vi "PH_PSDBWriter.write Dataset.vi"(1 "PSDB Credentials":T1={"PW"="N/A", "ID"="N/A", "DS"="N/A"}, 2 "Shot #":i32, 3 "Instance ID":i32, 4 "Data to write to PSDB":T2, 5 "error in (no error)":errorcluster) -> (19 "error out":errorcluster)   [LabVIEW 2014, in "PH_PSDBWriter.lvlib"]
uses:
  PH_PSDBWriter.lvlib
  PH_PSDBWriter.PSDB Dataset.ctl
  PH_PSDBWriter.2D dataset.ctl
  CSlibraries-extern/psdb_lv/PSDB_AxisDescription.ctl
  PH_PSDBWriter.Boolean dataset.ctl
  PH_PSDBWriter.Image dataset.ctl
  <vilib>/vision/Image Controls.llb/IMAQ Image.ctl
  PH_PSDBWriter.Numeric dataset.ctl
  PH_PSDBWriter.String dataset.ctl
  PH_Common/Connection/PH_Connection.PSDB Credentials.ctl
  CSlibraries-extern/psdb_lv/PSDB_SetInstanceValue(2dData).vi
  CSlibraries-extern/psdb_lv/PSDB_SetInstanceValue(Boolean).vi
  CSlibraries-extern/psdb_lv/PSDB_SetInstanceValue(Image).vi
  CSlibraries-extern/psdb_lv/PSDB_SetInstanceValue(Numeric).vi
  CSlibraries-extern/psdb_lv/PSDB_SetInstanceValue(String).vi
  CSlibraries-extern/psdb_lv/PSDB.lvlib
  PH_Common/PH_Common.lvlib
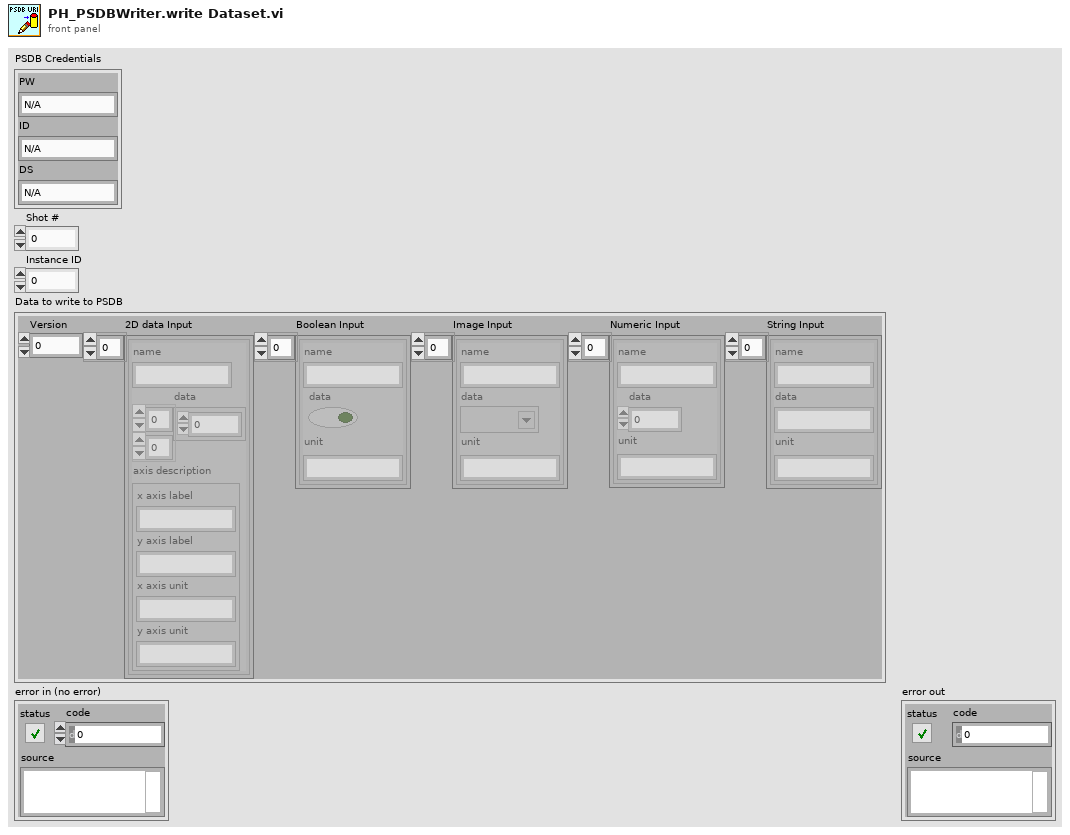
[diagram p1: front panel]
types:
  T1 = typedef "PH_Common.lvlib/PH_Connection.PSDB Credentials.ctl" = cluster{"PW":string, "ID":string, "DS":string}
  T2 = typedef "PH_PSDBWriter.lvlib/PH_PSDBWriter.PSDB Dataset.ctl" = cluster{"Version":i32, "2D data Input":T3[], "Boolean Input":T5[], "Image Input":T6[], "Numeric Input":T8[], "String Input":T9[]}
  T3 = typedef "PH_PSDBWriter.lvlib/PH_PSDBWriter.2D dataset.ctl" = cluster{"name":string, "data":dbl[][], "axis description":T4}
  T4 = typedef "PSDB.lvlib/PSDB_AxisDescription.ctl" = cluster{"x axis label":string, "y axis label":string, "x axis unit":string, "y axis unit":string}
  T5 = typedef "PH_PSDBWriter.lvlib/PH_PSDBWriter.Boolean dataset.ctl" = cluster{"name":string, "data":bool, "unit":string}
  T6 = typedef "PH_PSDBWriter.lvlib/PH_PSDBWriter.Image dataset.ctl" = cluster{"name":string, "data":T7, "unit":string}
  T7 = typedef "IMAQ Image.ctl" = refnum<image>
  T8 = typedef "PH_PSDBWriter.lvlib/PH_PSDBWriter.Numeric dataset.ctl" = cluster{"name":string, "data":dbl, "unit":string}
  T9 = typedef "PH_PSDBWriter.lvlib/PH_PSDBWriter.String dataset.ctl" = cluster{"name":string, "data":string, "unit":string}
  T10 = typedef "NI_Database_API.lvlib/Conn ObjectReference.ctl" = refnum<k1>
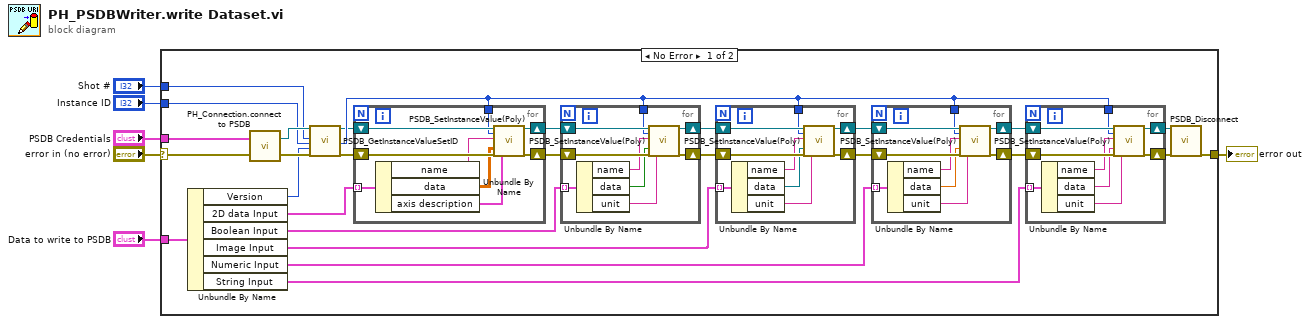
[diagram p0: block diagram]
diagram:
  n1 = case shown="No Error" "error in (no error)" {
    selector: "error in (no error)" -> [w8 w79]
    tunnel: [w33 w79] -> w6
    tunnel: "Shot #" -> [w17 _]
    tunnel: "Instance ID" -> [w16 _]
    tunnel: "Data to write to PSDB" -> [w15 _]
    tunnel: "PSDB Credentials" -> [w7 _]
    frame No Error {
      n2 = Unbundle By Name(w15) -> ("Version"=w9:i32, "2D data Input"=w10:T3[], "Boolean Input"=w11:T5[], "Image Input"=w12:T6[], "Numeric Input"=w13:T8[], "String Input"=w14:T9[])
      n3 = call "PH_Connection.connect to PSDB.vi"("error in"=w8, "PSDB Credentials"=w7) -> ("error out"=w18:errorcluster, "connection reference"=w19:T10)
      n4 = call "PSDB_GetInstanceValueSetID.vi"("connection reference"=w19, "shot_id"=w17, "instance_id"=w16, "version (0)"=w9, "error in (no error)"=w18) -> ("connection reference out"=w21:T10, "instancevalueset_id"=w31:i32, "error out"=w20:errorcluster)  [unwired: 12 in]
      n5 = for {
        tunnel: w31 -> [w74]
        shift-right: [w75] -> w32
        shift-left: w21 -> [w76]
        shift-right: [w77] -> w22
        shift-left: w20 -> [w78]
        tunnel: w10 -> [w73] mode=indexing
        n6 = Unbundle By Name(w73) -> ("name"=w72:string, "data"=w71:dbl[][], "axis description"=w70:T4)
        n7 = call-poly "PSDB_SetInstanceValue(Poly).vi"("connection reference"=w76, "instancevalueset_id"=w74, "name"=w72, "data"=w71, "error in (no error)"=w78, "axis description"=w70) -> ("connection reference out"=w75:T10, "error out"=w77:errorcluster)  [unwired: 12 in]
      }
      n8 = for {
        tunnel: w31 -> [w65]
        shift-right: [w66] -> w24
        shift-left: w32 -> [w67]
        shift-right: [w68] -> w23
        shift-left: w22 -> [w69]
        tunnel: w11 -> [w64] mode=indexing
        n9 = Unbundle By Name(w64) -> ("name"=w63:string, "data"=w62:bool, "unit"=w61:string)
        n10 = call-poly "PSDB_SetInstanceValue(Poly).vi"("connection reference"=w67, "instancevalueset_id"=w65, "name"=w63, "data"=w62, "error in (no error)"=w69, "unit"=w61) -> ("connection reference out"=w66:T10, "error out"=w68:errorcluster)  [unwired: 12 in]
      }
      n11 = for {
        tunnel: w31 -> [w56]
        shift-right: [w57] -> w25
        shift-left: w24 -> [w58]
        shift-right: [w59] -> w26
        shift-left: w23 -> [w60]
        tunnel: w12 -> [w55] mode=indexing
        n12 = Unbundle By Name(w55) -> ("name"=w54:string, "data"=w53:T7, "unit"=w52:string)
        n13 = call-poly "PSDB_SetInstanceValue(Poly).vi"("connection reference"=w58, "instancevalueset_id"=w56, "name"=w54, "data"=w53, "error in (no error)"=w60, "unit"=w52) -> ("connection reference out"=w57:T10, "error out"=w59:errorcluster)  [unwired: 12 in]
      }
      n14 = for {
        tunnel: w31 -> [w47]
        shift-right: [w48] -> w28
        shift-left: w25 -> [w49]
        shift-right: [w50] -> w27
        shift-left: w26 -> [w51]
        tunnel: w13 -> [w46] mode=indexing
        n15 = Unbundle By Name(w46) -> ("name"=w45:string, "data"=w44:dbl, "unit"=w43:string)
        n16 = call-poly "PSDB_SetInstanceValue(Poly).vi"("connection reference"=w49, "instancevalueset_id"=w47, "name"=w45, "data"=w44, "error in (no error)"=w51, "unit"=w43) -> ("connection reference out"=w48:T10, "error out"=w50:errorcluster)  [unwired: 12 in]
      }
      n17 = for {
        tunnel: w31 -> [w38]
        shift-right: [w39] -> w30
        shift-left: w28 -> [w40]
        shift-right: [w41] -> w29
        shift-left: w27 -> [w42]
        tunnel: w14 -> [w37] mode=indexing
        n18 = Unbundle By Name(w37) -> ("name"=w36:string, "data"=w35:string, "unit"=w34:string)
        n19 = call-poly "PSDB_SetInstanceValue(Poly).vi"("connection reference"=w40, "instancevalueset_id"=w38, "name"=w36, "data"=w35, "error in (no error)"=w42, "unit"=w34) -> ("connection reference out"=w39:T10, "error out"=w41:errorcluster)  [unwired: 12 in]
      }
      n20 = call "PSDB_Disconnect.vi"("connection reference"=w30, "error in (no error)"=w29) -> ("error out"=w33:errorcluster)  [unwired: 17 in]
    }
    frame Error {
    }
  }
  "error out" <- w6
